vi "is Packet Timeout.vi"(11 "port_num":i32) -> (3 "function return":u8)   [LabVIEW 2015, in "dxl_x86_c.lvlib"]
doc: "WINDECLSPEC uint8_t isPacketTimeout (int port_num);"
uses:
  dxl_x86_c.lvlib
  dxl_x86_c.dll
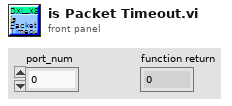
[diagram p1: front panel]
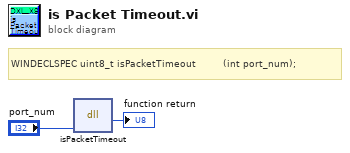
[diagram p0: block diagram]
diagram:
  # "WINDECLSPEC uint8_t isPacketTimeout         (int port_num);"
  n1 = dll-call lib="C:/Users/Platform/Desktop/LabVIEW/dxl_x86_c.lvlib/dxl_x86_c.*" fn="isPacketTimeout"("port_num"="port_num") -> (→"function return":u8)  [unwired: 4 in, 2 out]
